vi "New Nested.vi"(8 "error in (no error)":errorcluster, 11 "caller actor in":refnum<class "Actor.lvclass">) -> (0 "error out":errorcluster, 2 "normal log":refnum<class "Normal Log.lvclass">, 3 "caller actor out":refnum<class "Actor.lvclass">)   [LabVIEW 2020, in "Normal Log.lvlib" / "Normal Log.lvclass"]
uses:
  Normal Log.lvclass
  <vilib>/ActorFramework/Actor/Actor.lvclass
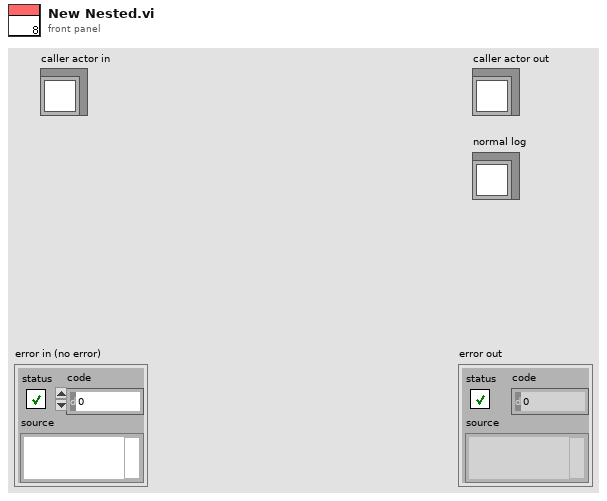
[diagram p1: front panel]
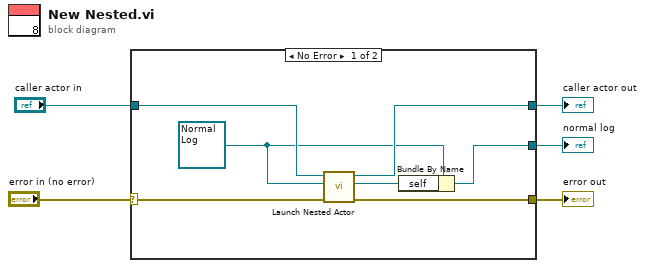
[diagram p0: block diagram]
diagram:
  n1 = case shown="No Error" "error in (no error)" {
    selector: "error in (no error)" -> [w12 w14]
    tunnel: [w8 w14] -> w4
    tunnel: [w9 _] -> w3
    tunnel: "caller actor in" -> [w11 w13]
    tunnel: [w7 w13] -> w1
    frame No Error {
      w6 = refnum<class "Normal Log.lvclass"> refnum ("Normal Log in")
      n2 = call <vilib>:"Launch Nested Actor.vi"("error in (no error)"=w12, "Nested Actor"=w6, "Caller Actor in"=w11) -> ("error out"=w8:errorcluster, "Nested Actor's Enqueuer"=w10:refnum<class "Message Enqueuer.lvclass">, "Caller Actor out"=w7:refnum<class "Actor.lvclass">)  [unwired: 6 in]
      n3 = Bundle By Name(cluster=w6, "self"=w10) -> (w9:refnum<class "Normal Log.lvclass">)
    }
    frame Error {
    }
  }
  "error out" <- w4
  "normal log" <- w3
  "caller actor out" <- w1
